vi "Save Known Packages.vi"(8 "error in (no error)":errorcluster, 11 "Package Array from File":T1[](array[typedef])) -> (0 "error out":errorcluster, 1 "Success?":bool)   [LabVIEW 2019, in "Project.Dependencies Finder.lvlib" / "Dependency Source_VIPM.lvclass"]
doc: "Load package info from file."
uses:
  Dependency Source_VIPM.lvclass
  Ctl/Ctl_Package Identifier Cluster.ctl
  <vilib>/Utility/file.llb/Write Delimited Spreadsheet (string).vi
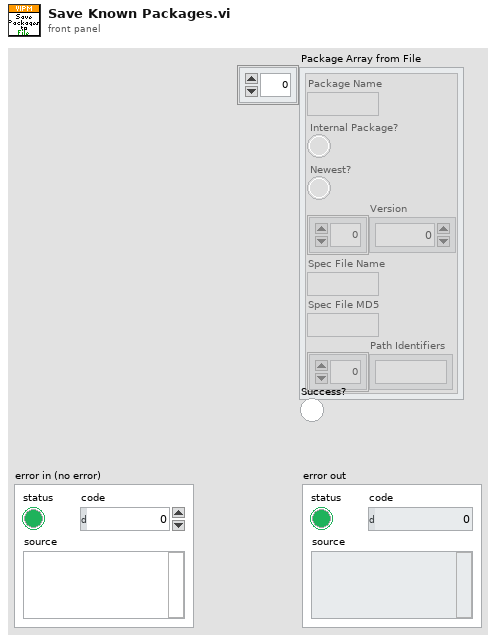
[diagram p1: front panel]
types:
  T1 = typedef "Project.Dependencies Finder.lvlib/Dependency Source_VIPM.lvclass/Ctl_Package Identifier Cluster.ctl" = cluster{"Package Name":string, "Internal Package?":bool, "Newest?":bool, "Version":i32[], "Spec File Name":string, "Spec File MD5":string, "Path Identifiers":string[]}
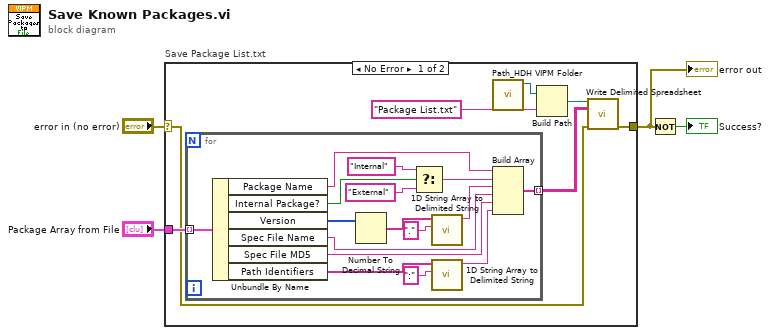
[diagram p0: block diagram]
diagram:
  n1 = case "Save Package List.txt" shown="No Error" "error in (no error)" {
    selector: "error in (no error)" -> [w9 w28]
    tunnel: "Package Array from File" -> [w11 _]
    tunnel: [w8 w28] -> w2
    frame No Error {
      n2 = for {
        tunnel: w11 -> [w27] mode=indexing
        tunnel: [w20] -> w10 mode=indexing
        n3 = Unbundle By Name(w27) -> ("Package Name"=w26:string, "Internal Package?"=w17:bool, "Version"=w15:i32[], "Spec File Name"=w25:string, "Spec File MD5"=w24:string, "Path Identifiers"=w23:string[])
        n4 = Number To Decimal String(number=w15) -> (decimal integer string=w14:string[])  [unwired: 1 in]
        n5 = Select(t="Internal", s=w17, f="External") -> (s? t:f=w16:string)
        n6 = call <vilib>:"1D String Array to Delimited String.vi"("delimiter"=".", "string array"=w14) -> ("delimited string"=w12:string)  [unwired: 9 in]
        n7 = call <vilib>:"1D String Array to Delimited String.vi"("delimiter"=":", "string array"=w23) -> ("delimited string"=w21:string)  [unwired: 9 in]
        n8 = Build Array(w26, w16, w12, w25, w24, w21) -> (w20:string[])
      }
      n9 = call "Path_HDH VIPM Folder.vi"() -> ("HDH\\VIPM path"=w7:path)  [unwired: 10 in, 1 out]
      n10 = Build Path(base path=w7, name or relative path="Package List.txt") -> (appended path=w5:path)
      n11 = call-poly <vilib>:"Write Delimited Spreadsheet.vi"("file path (dialog if empty)"=w5, "2D data"=w10, "error in (no error)"=w9) -> ("error out"=w8:errorcluster)  [unwired: 11 in, 1 out]
    }
    frame Error {
    }
  }
  "error out" <- w2
  n12 = Not(x=w2) -> (.not. x?=→"Success?":bool)
